vi "Read.vi"(8 "error in (no error)":errorcluster, 11 "Numeric Variable in":refnum<class "Double Float.lvclass">) -> (0 "error out":errorcluster, 2 "Numeric":dbl, 3 "Numeric Variable out":refnum<class "Double Float.lvclass">)   [LabVIEW 2021, in "Variable.lvlib" / "Double Float.lvclass"]
uses:
  Double Float.lvclass
  Double Float.lvclass/Double Float.ctl
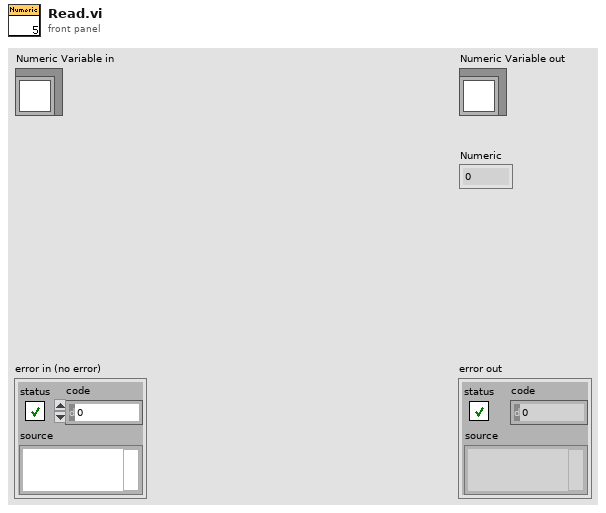
[diagram p1: front panel]
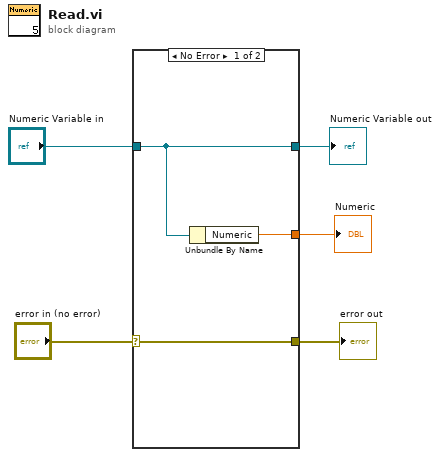
[diagram p0: block diagram]
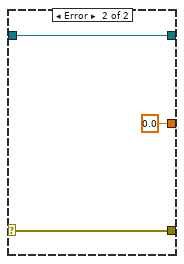
[diagram p2: hidden frame]
diagram:
  n1 = case shown="No Error" "error in (no error)" {
    selector: "error in (no error)" -> [w6 w10]
    tunnel: "Numeric Variable in" -> [w8 w11]
    tunnel: [w8 w11] -> w4
    tunnel: [w7 0.0 ("Numeric")] -> w3
    tunnel: [w6 w10] -> w2
    frame No Error {
      n2 = Unbundle By Name(w8) -> ("Numeric"=w7:dbl)
    }
    frame Error {
    }
  }
  "error out" <- w2
  "Numeric Variable out" <- w4
  "Numeric" <- w3
